vi "Read Keytap.vi"(7 "Error In":errorcluster, 9 "Key Tap Thresh":sgl=55.0 caption="Key Tap Threshold", 10 "Leap Handle In":T1) -> (0 "Error Out":errorcluster, 1 "PinchStrength":sgl, 2 "Key tap":string[](array[string]), 3 "Leap Handle Out":T1, 4 "Tip Velocity Module":dbl[](array[numeric]), 5 "Index Array":bool[](array[boolean]))   [LabVIEW 2014]
doc: "<b>Leap Read</b> requests and parses a <b>Frame</b> of data from the Leap Motion Controller. All the data associated with the Frame is organized into a LabVIEW cluster for accessibility.\n\nSpecifics about the data in the Frame cluster can be found by going to <b>Help » Leap Motion Controller Help</b> inside of LabVIEW"
uses:
  Typedef 2.0/Leap Handle.ctl
  C:/Users/Frax/Desktop/Progetti avanzati Labview/Smart Wristband/Smart Wristband/Leap Motion VIs 2.0/LeapCSharp.NET4.0.dll
  LeapCSharp.NET4.0.dll
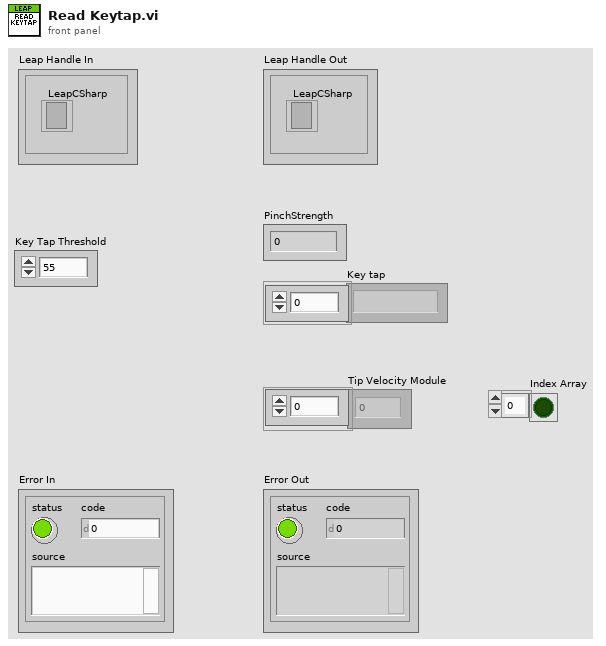
[diagram p1: front panel]
types:
  T1 = typedef "Leap Handle.ctl" = cluster{"LeapCSharp":refnum<k24>}
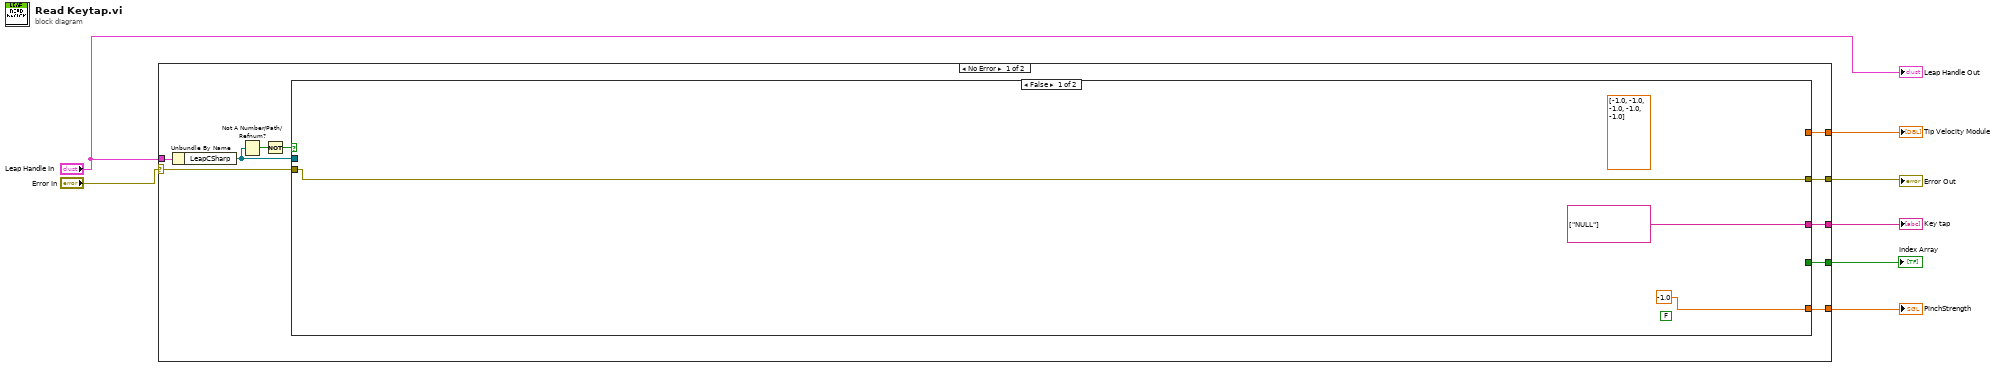
[diagram p0: block diagram]
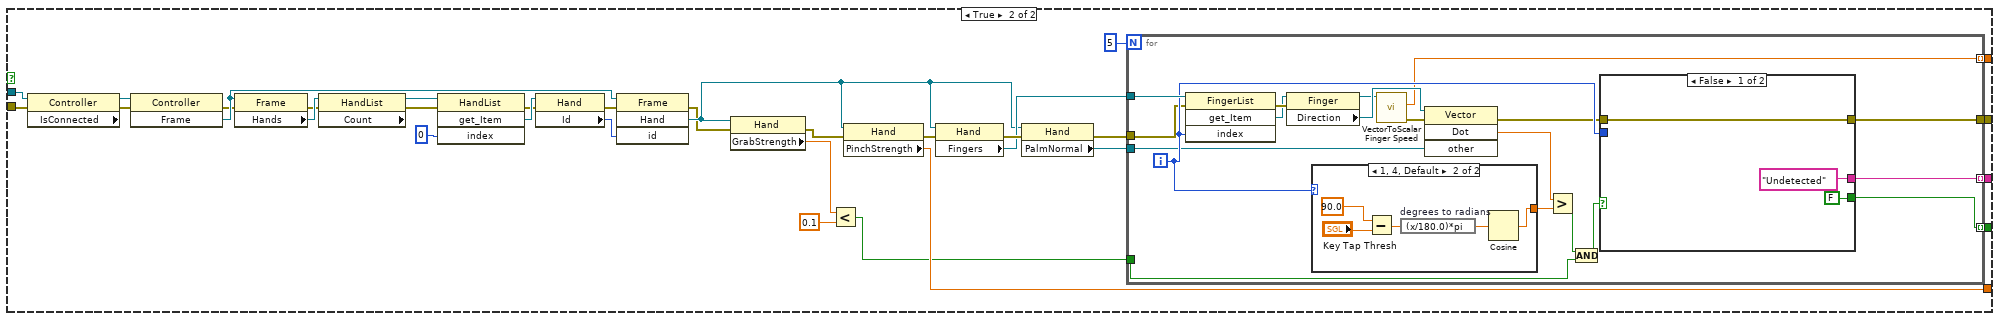
[diagram p2: hidden frame]
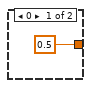
[diagram p3: hidden frame]
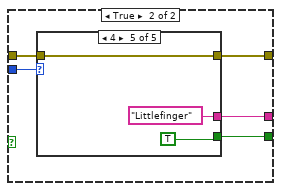
[diagram p4: hidden frame]
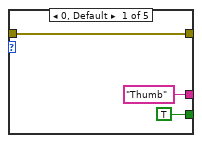
[diagram p5: hidden frame]
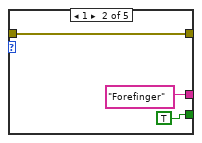
[diagram p6: hidden frame]
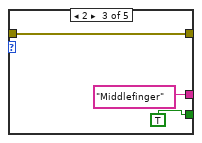
[diagram p7: hidden frame]
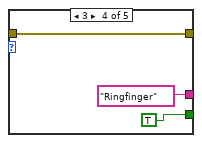
[diagram p8: hidden frame]
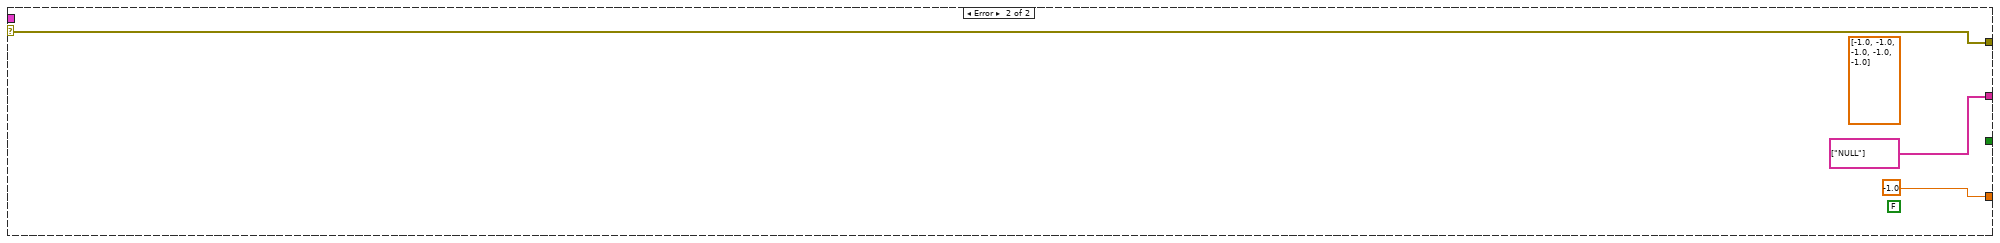
[diagram p9: hidden frame]
diagram:
  n1 = case shown="No Error" "Error In" {
    selector: "Error In" -> [w16 w102]
    tunnel: "Leap Handle In" -> [w17 _]
    tunnel: [w15 w102] -> w4
    tunnel: [w11 string[] ["NULL"]] -> w5
    tunnel: [w10 sgl -1.0 ("PinchStrength")] -> w3
    tunnel: [w9 _] -> w2
    tunnel: [w8 _] -> w1
    frame No Error {
      n2 = Unbundle By Name(w17) -> ("LeapCSharp"=w12:refnum<k24>)
      n3 = Not A Number/Path/Refnum?(number/path/refnum=w12) -> (NaN/Path/Refnum?=w14:bool)
      n4 = Not(x=w14) -> (.not. x?=w13:bool)
      n5 = case shown="False" w13 {
        tunnel: w16 -> [w19 w52]
        tunnel: [w19 w32] -> w15
        tunnel: w12 -> [_ w49]
        tunnel: [string[] ["NULL"] w34] -> w11
        tunnel: [sgl -1.0 ("PinchStrength") w29] -> w10
        tunnel: [_ w28] -> w9
        tunnel: [_ w21] -> w8
        frame False {
          (unwired) sgl[] [-1.0, -1.0, -1.0, -1.0, -1.0]
          (unwired) FALSE ("IsConnected")
        }
        frame True {
          n6 = property class="Controller" props=["IsConnected"](reference=w49, error in=w52) -> (reference out=w51:refnum<k24>, error out=w50:errorcluster)  [unwired: 1 out]
          n7 = invoke class="Controller" method="Frame"(reference=w51, error in=w50) -> (error out=w42:errorcluster, "Frame"=w43:refnum<k24>)  [unwired: 1 in, 1 out]
          n8 = property class="Frame"(reference=w43, error in=w42) -> (error out=w41:errorcluster, "Hands"=w48:refnum<k24>)  [unwired: 1 out]
          n9 = property class="HandList" props=["Count"](reference=w48, error in=w41) -> (reference out=w47:refnum<k24>, error out=w40:errorcluster)  [unwired: 1 out]
          n10 = invoke class="HandList" method="get_Item"(reference=w47, error in=w40, "index"=0) -> (error out=w39:errorcluster, "get_Item"=w45:refnum<k24>)  [unwired: 1 in, 2 out]
          n11 = property class="Hand"(reference=w45, error in=w39) -> (error out=w38:errorcluster, "Id"=w44:i32)  [unwired: 1 out]
          n12 = invoke class="Frame" method="Hand"(reference=w43, error in=w38, "id"=w44) -> (error out=w26:errorcluster, "Hand"=w27:refnum<k24>)  [unwired: 1 in, 2 out]
          n13 = property class="Hand"(reference=w27, error in=w26) -> (error out=w25:errorcluster, "GrabStrength"=w23:sgl)  [unwired: 1 out]
          n14 = Less?(x=w23, y=0.1) -> (x < y?=w22:bool)
          n15 = property class="Hand"(reference=w27, error in=w25) -> (error out=w31:errorcluster, "PinchStrength"=w29:sgl)  [unwired: 1 out]
          n16 = property class="Hand"(reference=w27, error in=w31) -> (error out=w36:errorcluster, "Fingers"=w30:refnum<k24>)  [unwired: 1 out]
          n17 = property class="Hand"(reference=w27, error in=w36) -> (error out=w33:errorcluster, "PalmNormal"=w35:refnum<k24>)  [unwired: 1 out]
          n18 = for {
            N: 5 -> [_]
            tunnel: w30 -> [w71]
            tunnel: w35 -> [w64]
            tunnel: [w70] -> w34 mode=indexing
            tunnel: w33 -> [w68]
            tunnel: [w62] -> w32
            tunnel: [w60] -> w28 mode=indexing
            tunnel: w22 -> [w58]
            tunnel: [w53] -> w21 mode=indexing
            i -> [w69]
            n19 = invoke class="FingerList" method="get_Item"(reference=w71, error in=w68, "index"=w69) -> (error out=w67:errorcluster, "get_Item"=w61:refnum<k24>)  [unwired: 1 in, 2 out]
            n20 = property class="Finger"(reference=w61, error in=w67) -> (reference out=w54:refnum<k24>, "Direction"=w65:refnum<k24>)  [unwired: 1 out]
            n21 = case shown="1, 4, Default" w69 {
              tunnel: [sgl 0.5 ("Altre Dita Key Tap Threshold") w75] -> w66
              frame 0 {
              }
              frame 1, 4, Default {
                n22 = Subtract(x=90.0, y="Key Tap Thresh") -> (x-y=w74:dbl)
                n23 = expression code="(x/180.0)*pi" "degrees to radians"(w74) -> (w73:dbl)
                n24 = Cosine(x=w73) -> (cos(x)=w75:dbl)
              }
            }
            n25 = call "VectorToScalar Finger Speed.vi"("reference"=w54) -> ("error out"=w59:errorcluster, "sqrt(x)"=w60:sgl)  [unwired: 9 in]
            n26 = invoke class="Vector" method="Dot"(reference=w65, error in=w59, "other"=w64) -> (error out=w63:errorcluster, "Dot"=w55:sgl)  [unwired: 1 in, 2 out]
            n27 = Greater?(x=w55, y=w66) -> (0:w57:bool)
            n28 = And(x=w57, y=w58) -> (x .and. y?=w56:bool)
            n29 = case shown="False" w56 {
              tunnel: ["Undetected" w85] -> w70
              tunnel: w69 -> [_ w82]
              tunnel: w63 -> [w79 w84]
              tunnel: [w79 w83] -> w62
              tunnel: [FALSE w81] -> w53
              frame False {
              }
              frame True {
                n30 = case shown="4" w82 {
                  tunnel: ["Thumb" "Forefinger" "Middlefinger" "Ringfinger" "Littlefinger"] -> w85
                  tunnel: w84 -> [w87 w90 w93 w96 w99]
                  tunnel: [w87 w90 w93 w96 w99] -> w83
                  tunnel: [TRUE TRUE TRUE TRUE TRUE] -> w81
                  frame 0, Default {
                  }
                  frame 1 {
                  }
                  frame 2 {
                  }
                  frame 3 {
                  }
                  frame 4 {
                  }
                }
              }
            }
          }
        }
      }
    }
    frame Error {
      (unwired) sgl[] [-1.0, -1.0, -1.0, -1.0, -1.0]
      (unwired) FALSE ("IsConnected")
    }
  }
  "Error Out" <- w4
  "Key tap" <- w5
  "PinchStrength" <- w3
  "Tip Velocity Module" <- w2
  "Index Array" <- w1
  "Leap Handle Out" <- "Leap Handle In"
